vi "Show Hide Window.vi"(6 "Close VI Reference? (T)":bool=TRUE, 8 "error in (no error)":errorcluster, 9 "Method (Show Window)":T1, 10 "VI Reference (Calling VI)":refnum<vi>) -> (0 "error out":errorcluster, 2 "VI Reference":refnum<vi>)   [LabVIEW 2011]
doc: "This VI is used for managing a LabVIEW front panel, based on the VI reference passed in. If a reference is not passed in, the code will operate on the Calling VI.\n\n-------------\nDeveloped by Brian Hoover (hooovahh)"
uses:
  Show Hide Window Methods.ctl
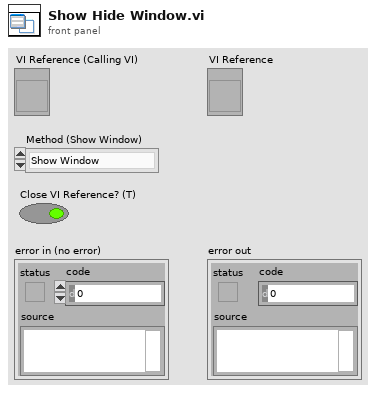
[diagram p1: front panel]
types:
  T1 = typedef "Show Hide Window Methods.ctl" = enum16{"Show Window", "Hide Window", "Close Window", "Minimize Window", "Maximize Window"}
  T2 = enum32{"Invalid", "Standard", "Closed", "Hidden", "Minimized", "Maximized"}
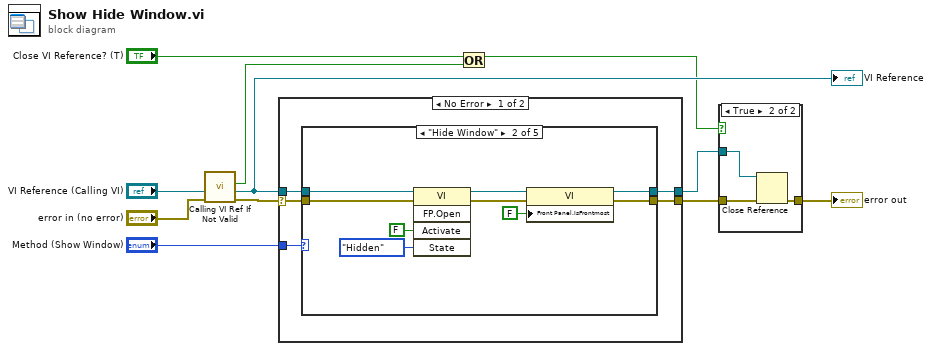
[diagram p0: block diagram]
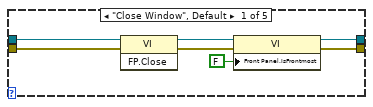
[diagram p3: hidden frame]
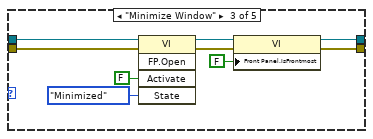
[diagram p4: hidden frame]
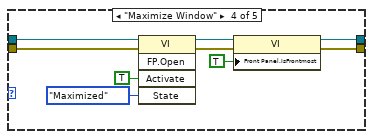
[diagram p5: hidden frame]
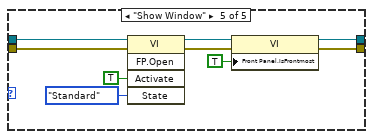
[diagram p6: hidden frame]
diagram:
  n1 = call "Calling VI Ref If Not Valid.vi"("error in (no error)"="error in (no error)", "VI Reference"="VI Reference (Calling VI)") -> ("error out"=w8:errorcluster, "Valid VI Ref"=w7:refnum<vi>, "New Reference Opened"=w1:bool)  [unwired: 7 in]
  "VI Reference" <- w7
  n2 = case shown="No Error" w8 {
    selector: w8 -> [w14 w60]
    tunnel: w7 -> [w16 w61]
    tunnel: "Method (Show Window)" -> [w15 _]
    tunnel: [w13 w61] -> w5
    tunnel: [w12 w60] -> w6
    frame No Error {
      n3 = case shown="\"Hide Window\"" w15 {
        tunnel: w16 -> [w20 w29 w38 w47 w54]
        tunnel: w14 -> [w19 w28 w37 w46 w53]
        tunnel: [w17 w26 w35 w44 w52] -> w12
        tunnel: [w18 w27 w36 w45 w51] -> w13
        frame "Close Window", Default {
          n4 = invoke class="VI" method="FP.Close"(reference=w20, error in=w19) -> (reference out=w22:refnum<vi>, error out=w21:errorcluster)  [unwired: 1 in, 1 out]
          n5 = property class="VI"(reference=w22, error in=w21, "Front Panel.IsFrontmost"=FALSE ("Front Panel Window:Is Frontmost")) -> (reference out=w18:refnum<vi>, error out=w17:errorcluster)
        }
        frame "Hide Window" {
          n6 = invoke class="VI" method="FP.Open"(reference=w29, error in=w28, "Activate"=FALSE ("Activate?"), "State"=T2."Hidden") -> (reference out=w31:refnum<vi>, error out=w30:errorcluster)  [unwired: 1 in, 3 out]
          n7 = property class="VI"(reference=w31, error in=w30, "Front Panel.IsFrontmost"=FALSE ("Front Panel Window:Is Frontmost")) -> (reference out=w27:refnum<vi>, error out=w26:errorcluster)
        }
        frame "Minimize Window" {
          n8 = invoke class="VI" method="FP.Open"(reference=w38, error in=w37, "Activate"=FALSE ("Activate?"), "State"=T2."Minimized") -> (reference out=w40:refnum<vi>, error out=w39:errorcluster)  [unwired: 1 in, 3 out]
          n9 = property class="VI"(reference=w40, error in=w39, "Front Panel.IsFrontmost"=FALSE ("Front Panel Window:Is Frontmost")) -> (reference out=w36:refnum<vi>, error out=w35:errorcluster)
        }
        frame "Maximize Window" {
          n10 = invoke class="VI" method="FP.Open"(reference=w47, error in=w46, "Activate"=TRUE ("Activate?"), "State"=T2."Maximized") -> (reference out=w49:refnum<vi>, error out=w48:errorcluster)  [unwired: 1 in, 3 out]
          n11 = property class="VI"(reference=w49, error in=w48, "Front Panel.IsFrontmost"=TRUE ("Front Panel Window:Is Frontmost")) -> (reference out=w45:refnum<vi>, error out=w44:errorcluster)
        }
        frame "Show Window" {
          n12 = invoke class="VI" method="FP.Open"(reference=w54, error in=w53, "Activate"=TRUE ("Activate?"), "State"=T2."Standard") -> (reference out=w56:refnum<vi>, error out=w55:errorcluster)  [unwired: 1 in, 3 out]
          n13 = property class="VI"(reference=w56, error in=w55, "Front Panel.IsFrontmost"=TRUE ("Front Panel Window:Is Frontmost")) -> (reference out=w51:refnum<vi>, error out=w52:errorcluster)
        }
      }
    }
    frame Error {
    }
  }
  n14 = Or(x="Close VI Reference? (T)", y=w1) -> (x .or. y?=w2:bool)
  n15 = case shown="True" w2 {
    tunnel: w5 -> [_ w65]
    tunnel: w6 -> [w62 w64]
    tunnel: [w62 w63] -> w4
    frame False {
    }
    frame True {
      n16 = Close Reference(reference=w65, error in (no error)=w64) -> (error out=w63:errorcluster)
    }
  }
  "error out" <- w4
